vi "JoystickDataTest.vi"() -> ()   [LabVIEW 2016]
uses:
  JoystickData/JoystickData.ctl
panel:
  in  "ControllerData":T1
  in  "GyroAngle":dbl
  out "SwerveCommands":dbl[](array[numeric])
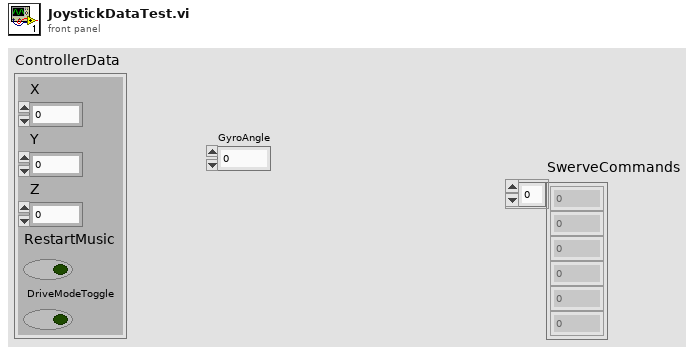
[diagram p1: front panel]
types:
  T1 = typedef "JoystickData.ctl" = cluster{"X":dbl, "Y":dbl, "Z":dbl, "RestartMusic":bool, "DriveModeToggle":bool}
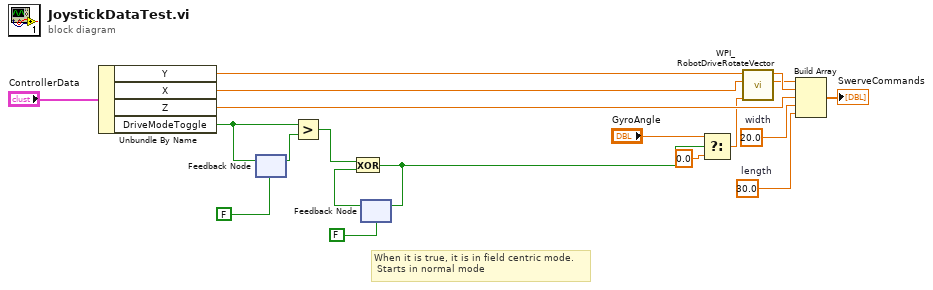
[diagram p0: block diagram]
diagram:
  w17 = 30.0  # length
  w18 = 20.0  # width
  # "When it is true, it is in field centric mode.\n Starts in normal mode"
  n1 = Unbundle By Name("ControllerData") -> ("Y"=w16:dbl, "X"=w15:dbl, "Z"=w12:dbl, "DriveModeToggle"=w10:bool)
  n2 = feedback #1(FALSE ("DriveModeToggle")) -> (w9:bool)
  n3 = feedback-in #1(w10) -> ()
  n4 = Greater?(x=w10, y=w9) -> (0:w8:bool)
  n5 = feedback #2(FALSE) -> (w6:bool)
  n6 = Exclusive Or(1:w6, 2:w8) -> (0:w7:bool)
  n7 = feedback-in #2(w7) -> ()
  n8 = Select(t="GyroAngle", s=w7, f=0.0 ("t")) -> (s? t:f=w3:dbl)
  n9 = call <vilib>:"WPI_RobotDriveRotateVector.vi"("Angle"=w3, "X"=w15, "Y"=w16) -> ("X'"=w13:dbl, "Y'"=w14:dbl)  [unwired: 7 out]
  n10 = Build Array(w13, w14, w12, w18, w17) -> (→"SwerveCommands":dbl[])
